vi "SCPI.vi"(4 "error in":T13, 7 "Command":string) -> (0 "error out":T13, 3 "Response":T11)   [LabVIEW 2018]
uses:
  MOKO_LabViewLibrary/MokoLowLevel/MokoLowLovelControl/MLLC_Error.ctl
  MOKO_LabViewLibrary/MokoLowLevel/MokoLowLovelControl/MLLC_Mode.ctl
  MOKO_LabViewLibrary/MokoLowLevel/MokoLowLovelControl/MLLC_Response.ctl
  MOKO_LabViewLibrary/MokoLowLevel/MokoLowLovelControl/MLLC_ConnectCluster.ctl
  MOKO_LabViewLibrary/MokoLowLevel/MokoLowLovelControl/MLLC_InterfaceType.ctl
  MOKO_LabViewLibrary/MokoLowLevel/MokoLowLovelControl/MLLC_OpenedSession.ctl
  MOKO_LabViewLibrary/MokoLowLevel/MokoLowLovelControl/MLLC_InterfaceSettings.ctl
  MOKO_LabViewLibrary/MokoLowLevel/MokoLowLovelControl/MLLC_InterfaceKind.ctl
  MOKO_LabViewLibrary/MokoLowLevel/MokoLowLovelControl/MLLC_DriverName.ctl
  MOKO_LabViewLibrary/MokoLowLevel/MokoLowLovelControl/MLLC_ErrorCode.ctl
  MOKO_LabViewLibrary/MokoLowLevel/MokoLowLovelControl/MLLC_ResponseInit.ctl
  MOKO_LabViewLibrary/MokoLowLevel/MokoLowLovelControl/MLLC_Request.ctl
panel:
  in  "Request":T1="*IDN?"
  in  "Response Init":T2="SCPI"
  in  "Error Code":T3=5450
  in  "Driver Name":T4="SCPI"
  in  "Settings":T10={"Saved Data"=variant, "Permanent data"={"Connect"={"InterfaceType"=enum."VISA", "OpenedSession"="COM1", "InterfaceSettings"={"Interface"=enum."Ethernet", "EOS 4 read"=enum."LF (\\n)", "EOS 4 write"=enum."LF (\\n)", "TMO, ms"=10000, "Sett"=variant(cluster{"Baud Rate":u32, "Data Bits":u16, "Parity":u16, "Stop Bits":u16, "Flow Control":u16, "Eho":bool} {"Baud Rate"=75, "Data Bits"=0, "Parity"=0, "Stop Bits"=0, "Flow Control"=0, "Eho"=FALSE})}}}}
  in  "Mode":T12=enum."Check"
  # "Example SCPI"
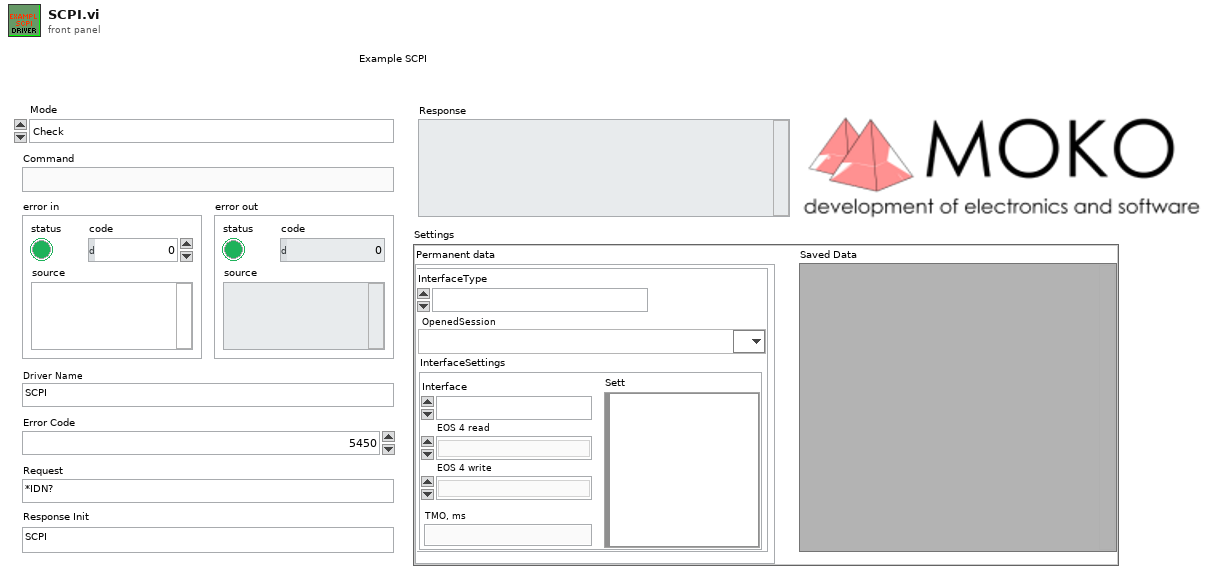
[diagram p1: front panel]
types:
  T1 = typedef "MLLC_Request.ctl" = string
  T2 = typedef "MLLC_ResponseInit.ctl" = string
  T3 = typedef "MLLC_ErrorCode.ctl" = u32
  T4 = typedef "MLLC_DriverName.ctl" = string
  T5 = typedef "MLLC_ConnectCluster.ctl" = cluster{"InterfaceType":T6, "OpenedSession":T7, "InterfaceSettings":T8}
  T6 = typedef "MLLC_InterfaceType.ctl" = enum16{"VISA", "Prologix USB-GPIB"}
  T7 = typedef "MLLC_OpenedSession.ctl" = refnum<visa-resource-name>
  T8 = typedef "MLLC_InterfaceSettings.ctl" = cluster{"Interface":T9, "EOS 4 read":enum16{"Default (=EOS 4 write)", "CR (\\r)", "LF (\\n)", "None"}, "EOS 4 write":enum16{"CR+LF (\\r\\n)", "CR (\\r)", "LF (\\n)", "None"}, "TMO, ms":i32, "Sett":variant}
  T9 = typedef "MLLC_InterfaceKind.ctl" = enum16{"RS232", "GPIB", "USB", "Ethernet", "another"}
  T10 = cluster{"Saved Data":variant, "Permanent data":cluster{"Connect":T5}}
  T11 = typedef "MLLC_Response.ctl" = string
  T12 = typedef "MLLC_Mode.ctl" = enum16{"get", "set", "close", "Init", "Check"}
  T13 = typedef "MLLC_Error.ctl" = errorcluster
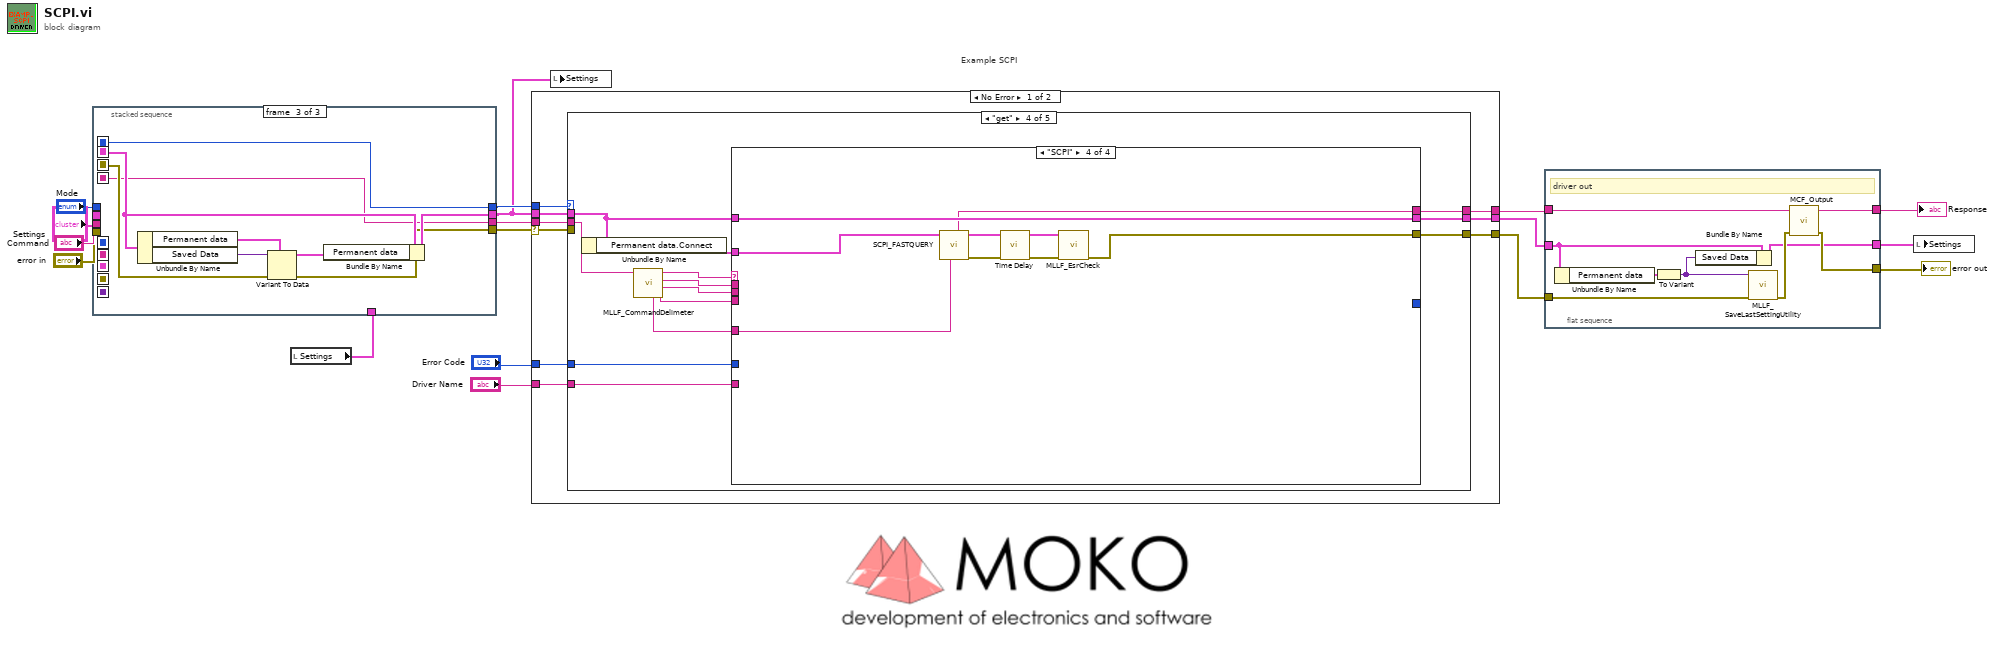
[diagram p0: block diagram]
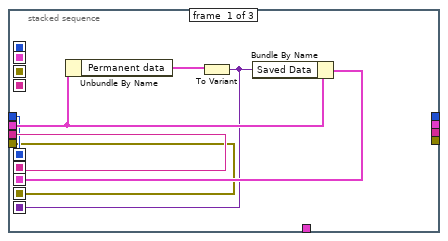
[diagram p2: hidden frame]
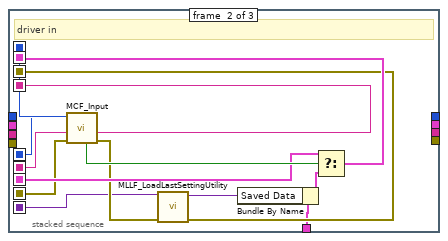
[diagram p3: hidden frame]
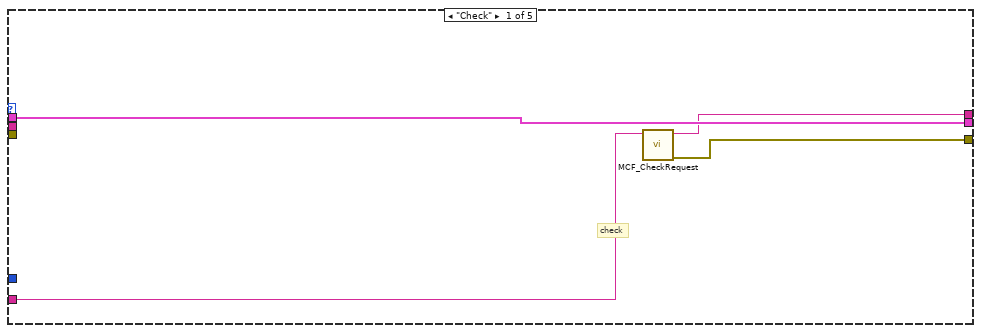
[diagram p4: hidden frame]
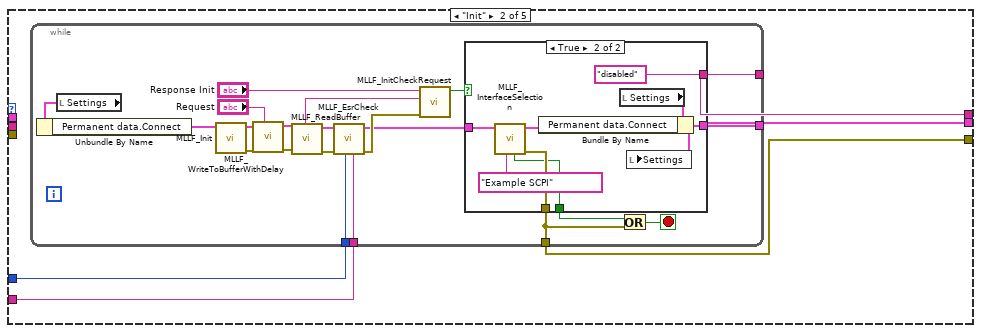
[diagram p5: hidden frame]
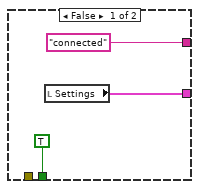
[diagram p6: hidden frame]
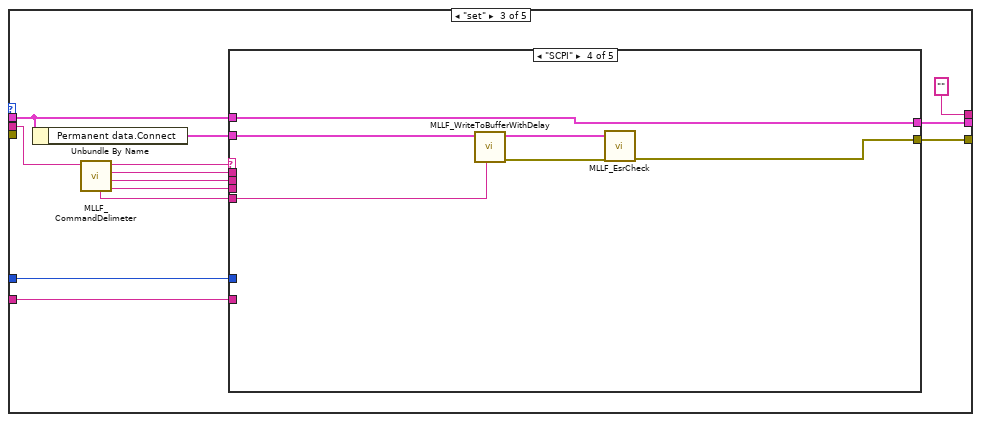
[diagram p7: hidden frame]
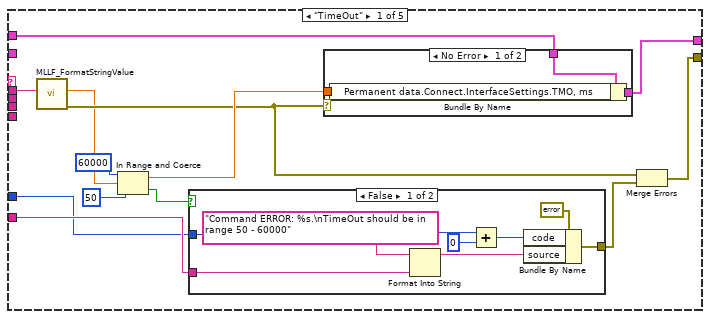
[diagram p8: hidden frame]
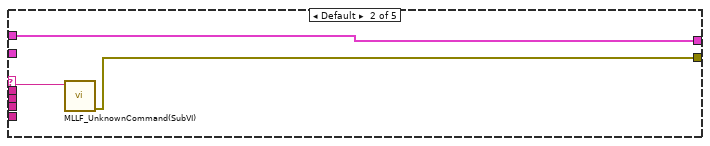
[diagram p11: hidden frame]
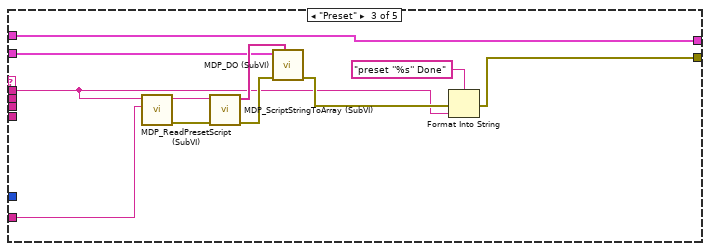
[diagram p12: hidden frame]
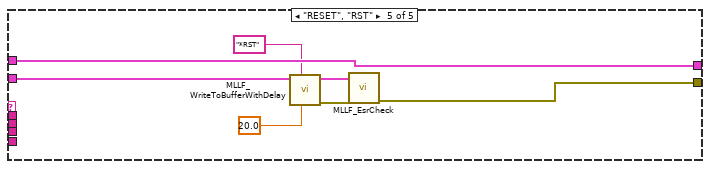
[diagram p13: hidden frame]
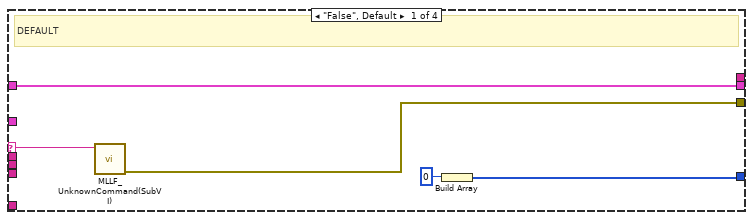
[diagram p14: hidden frame]
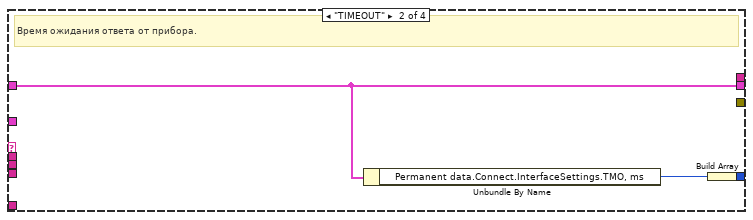
[diagram p15: hidden frame]
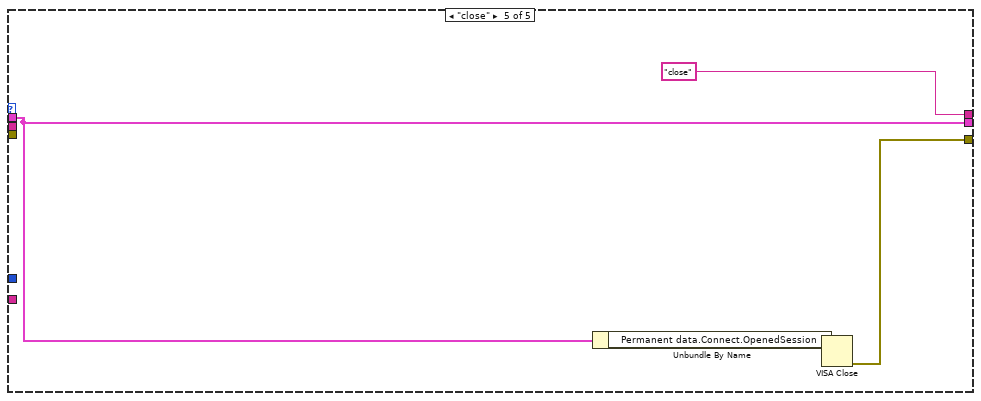
[diagram p17: hidden frame]
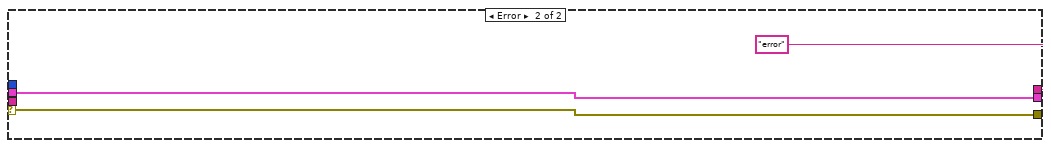
[diagram p18: hidden frame]
diagram:
  # "Example SCPI"
  n1 = local read "Settings"() -> (w7:T10)
  n2 = stacked-sequence {
    seq-local: [w20 _ _] -> [_ w36 _]
    seq-local: [w19 _ _] -> [_ w37 _]
    seq-local: [w22 _ _] -> [_ w32 _]
    seq-local: [w18 _ _] -> [_ w31 _]
    seq-local: [w21 _ _] -> [_ w27 _]
    seq-local: [_ w28 _] -> [_ _ w44]
    seq-local: [_ w38 _] -> [_ _ w41]
    seq-local: [_ w35 _] -> [_ _ w40]
    seq-local: [_ w34 _] -> [_ _ w45]
    tunnel: "Command" -> [w20 _ _]
    tunnel: "Mode" -> [w19 _ _]
    tunnel: "error in" -> [w18 _ _]
    tunnel: "Settings" -> [w23 _ _]
    tunnel: w7 -> [_ w26 _]
    tunnel: [_ _ w40] -> w9
    tunnel: [_ _ w43] -> w10
    tunnel: [_ _ w42] -> w8
    tunnel: [_ _ w41] -> w11
    frame #0 {
      n3 = Unbundle By Name(w23) -> ("Permanent data"=w24:cluster{"Connect":T5})
      n4 = To Variant(anything=w24) -> (Variant=w21:variant)
      n5 = Bundle By Name(cluster=w23, "Saved Data"=w21) -> (w22:T10)
    }
    frame #1 {
      # "driver in"
      n6 = call "MCF_Input.vi"("Error In"=w31, "Command in"=w36, "Mode in"=w37) -> ("Error Out"=w30:errorcluster, "Command out"=w35:string, "Mode out"=w38:T12, "Boolean"=w33:bool)  [unwired: 5 in]
      n7 = call "MLLF_LoadLastSettingUtility.vi"("Error In"=w30, "Save data in"=w27) -> ("Error Out"=w28:errorcluster, "Save data out"=w25:variant)  [unwired: 8 in]
      n8 = Bundle By Name(cluster=w26, "Saved Data"=w25) -> (w29:T10)
      n9 = Select(t=w32, s=w33, f=w29) -> (s? t:f=w34:T10)
    }
    frame #2 {
      n10 = Unbundle By Name(w45) -> ("Permanent data"=w46:cluster{"Connect":T5}, "Saved Data"=w39:variant)
      n11 = Variant To Data(error in=w44, type=w46, Variant=w39) -> (data=w47:cluster{"Connect":T5}, error out=w42:errorcluster)
      n12 = Bundle By Name(cluster=w45, "Permanent data"=w47) -> (w43:T10)
    }
  }
  n13 = case shown="No Error" w8 {
    selector: w8 -> [w52 w199]
    tunnel: [w54 w199] -> w4
    tunnel: w11 -> [w56 _]
    tunnel: [w55 "error" ("Output String")] -> w6
    tunnel: w9 -> [w53 _]
    tunnel: w10 -> [w49 w198]
    tunnel: "Error Code" -> [w51 _]
    tunnel: "Driver Name" -> [w50 _]
    tunnel: [w48 w198] -> w5
    frame No Error {
      n14 = case shown="\"get\"" w56 {
        tunnel: [w58 w63 "" ("Output String") w167 "close" ("Output String")] -> w55
        tunnel: [w57 w62 w103 w169 w195] -> w54
        tunnel: w53 -> [_ _ w110 w175 _]
        tunnel: w52 -> [_ _ _ _ _]
        tunnel: w51 -> [_ w65 w109 w172 _]
        tunnel: w50 -> [w59 w64 w106 w171 _]
        tunnel: w49 -> [w60 _ w108 w174 w194]
        tunnel: [w60 w61 w107 w173 w194] -> w48
        frame "Check" {
          # "check"
          # "Проверка подленности пользователя в соответствии с протоколом MD5."
          n15 = call "MCF_CheckRequest.vi"("Driver Name"=w59) -> ("Error Out"=w57:errorcluster, "Output String"=w58:string)  [unwired: 9 in]
        }
        frame "Init" {
          # "Тут проходит инициализация оборудования"
          n16 = while {
            tunnel: [w79] -> w62
            tunnel: w65 -> [w71]
            tunnel: w64 -> [w70]
            tunnel: [w76] -> w63
            tunnel: [w77] -> w61
            stop <- w78 stop-if-true
            n17 = local read "Settings"() -> (w82:T10)
            n18 = Unbundle By Name(w82) -> ("Permanent data.Connect"=w73:T5)
            n19 = call "MLLF_Init.vi"("DriverConnect in"=w73) -> ("Error Out"=w84:errorcluster, "DriverConnect out"=w83:T5)  [unwired: 7 in]
            n20 = call "MLLF_WriteToBufferWithDelay.vi"("Command"="Request", "Error In"=w84, "DriverConnect in"=w83) -> ("Error Out"=w86:errorcluster, "DriverConnect out"=w85:T5)  [unwired: 7 in]
            n21 = call "MLLF_ReadBuffer.vi"("Error In"=w86, "DriverConnect in"=w85) -> ("Error Out"=w68:errorcluster, "DriverConnect out"=w69:T5, "String"=w75:string)  [unwired: 6 in]
            n22 = call "MLLF_EsrCheck.vi"("Name"=w70, "Error code"=w71, "error in"=w68, "DriverConnect in"=w69) -> ("error out"=w67:T13, "DriverConnect out"=w66:T5)  [unwired: 6 in]
            n23 = call "MLLF_InitCheckRequest.vi"("error in (no error)"=w67, "Answer"=w75, "Response Init"="Response Init") -> ("Design"=w72:bool)  [unwired: 5 in, 3 out]
            n24 = case shown="True" w72 {
              tunnel: w66 -> [_ w96]
              tunnel: [TRUE w90] -> w80
              tunnel: [_ w97] -> w79
              tunnel: [w88 w92] -> w77
              tunnel: ["connected" "disabled"] -> w76
              frame False {
                n25 = local read "Settings"() -> (w88:T10)
              }
              frame True {
                n26 = call "MLLF_InterfaceSelection.vi"("Driver Name"="Example SCPI" ("String"), "DriverConnect in"=w96) -> ("error out"=w97:T13, "DriverConnect out"=w94:T5, "stop init?"=w90:bool)  [unwired: 7 in]
                n27 = local read "Settings"() -> (w93:T10)
                n28 = Bundle By Name(cluster=w93, "Permanent data.Connect"=w94) -> (w92:T10)
                n29 = local write "Settings"(w92) -> ()
              }
            }
            n30 = Or(x=w80, y=w79) -> (x .or. y?=w78:bool)
          }
        }
        frame "set" {
          # "Тут реализованы функции DriverSet"
          n31 = Unbundle By Name(w108) -> ("Permanent data.Connect"=w104:T5)
          n32 = call "MLLF_CommandDelimeter.vi"("command with param"=w110) -> ("param 3"=w99:string, "param 2"=w100:string, "param 1"=w101:string, "command"=w102:string, "Spit delimetre"=w98:string)  [unwired: 6 in]
          n33 = case shown="\"SCPI\"" w102 {
            selector: w102 -> [_ w137 _ _ _]
            tunnel: w108 -> [w113 w138 w139 w154 w162]
            tunnel: [w112 w138 w139 w154 w162] -> w107
            tunnel: w101 -> [w111 _ w142 _ _]
            tunnel: w109 -> [w115 _ _ _ _]
            tunnel: w106 -> [w116 _ w141 _ _]
            tunnel: [w114 w136 w140 w153 w161] -> w103
            tunnel: w104 -> [_ _ w143 w155 w160]
            tunnel: w100 -> [_ _ _ _ _]
            tunnel: w99 -> [_ _ _ _ _]
            tunnel: w98 -> [_ _ _ w150 _]
            frame "TimeOut" {
              n34 = call "MLLF_FormatStringValue.vi"("String Value"=w111) -> ("error out"=w118:T13, "number"=w117:dbl)  [unwired: 8 in, 1 out]
              n35 = In Range and Coerce(upper limit=60000, x=w117, lower limit=50) -> (coerced(x)=w121:dbl, In Range?=w119:bool)
              n36 = case shown="False" w119 {
                tunnel: [w130 _] -> w120
                tunnel: w115 -> [w129 _]
                tunnel: w116 -> [w128 _]
                frame False {
                  n37 = Format Into String(format string="Command ERROR: %s.\nTimeOut should be in range 50 - 60000", w128) -> (resulting string=w132:string)  [unwired: 2 in, 1 out]
                  n38 = Add(x=w129, y=0) -> (x+y=w133:T3)
                  n39 = Bundle By Name(cluster=errorcluster {"status"=TRUE, "code"=0, "source"=""} ("error out"), "code"=w133, "source"=w132) -> (w130:errorcluster)
                }
                frame True {
                }
              }
              n40 = case shown="No Error" w118 {
                tunnel: [w126 w127] -> w112
                tunnel: w113 -> [w125 w127]
                tunnel: w121 -> [w124 _]
                frame No Error {
                  n41 = Bundle By Name(cluster=w125, "Permanent data.Connect.InterfaceSettings.TMO, ms"=w124) -> (w126:T10)
                }
                frame Error {
                }
              }
              n42 = Merge Errors(w118, w120) -> (w114:errorcluster)
            }
            frame Default {
              n43 = call "MLLF_UnknownCommand(SubVI).vi"("Unknown command"=w137) -> ("error out"=w136:errorcluster)  [unwired: 10 in]
            }
            frame "Preset" {
              n44 = call "MDP_ReadPresetScript (SubVI).vi"("Driver Name"=w141, "String in"=w142) -> ("Error Out"=w147:errorcluster, "String out"=w148:string)  [unwired: 8 in]
              n45 = call "MDP_ScriptStringToArray (SubVI).vi"("Error In"=w147, "String script"=w148) -> ("Error Out"=w149:errorcluster, "Array script"=w144:string[])  [unwired: 8 in]
              n46 = call "MDP_DO (SubVI).vi"("Array script"=w144, "Error in (no error)"=w149, "DriverConnect in"=w143) -> ("Error Out"=w145:errorcluster)  [unwired: 7 in, 1 out]
              n47 = Format Into String(format string="preset ''%s'' Done" ("Befor substring"), error in=w145, w142) -> (error out=w140:errorcluster)  [unwired: 1 in, 1 out]
            }
            frame "SCPI" {
              n48 = call "MLLF_WriteToBufferWithDelay.vi"("Command"=w150, "DriverConnect in"=w155) -> ("Error Out"=w151:errorcluster, "DriverConnect out"=w152:T5)  [unwired: 8 in]
              n49 = call "MLLF_EsrCheck.vi"("error in"=w151, "DriverConnect in"=w152) -> ("error out"=w153:T13)  [unwired: 8 in, 1 out]
            }
            frame "RESET", "RST" {
              n50 = call "MLLF_WriteToBufferWithDelay.vi"("Delay Time ( 0,05 s)"=20.0, "Command"="*RST" ("string"), "DriverConnect in"=w160) -> ("Error Out"=w158:errorcluster, "DriverConnect out"=w157:T5)  [unwired: 7 in]
              n51 = call "MLLF_EsrCheck.vi"("error in"=w158, "DriverConnect in"=w157) -> ("error out"=w161:T13)  [unwired: 8 in, 1 out]
            }
          }
        }
        frame "get" {
          # "Тут реализованы функции DriverGet"
          n52 = Unbundle By Name(w174) -> ("Permanent data.Connect"=w170:T5)
          n53 = call "MLLF_CommandDelimeter.vi"("command with param"=w175) -> ("param 3"=w164:string, "param 2"=w165:string, "param 1"=w166:string, "command"=w168:string, "Spit delimetre"=w163:string)  [unwired: 6 in]
          n54 = case shown="\"SCPI\"" w168 {
            selector: w168 -> [w177 _ _ _]
            tunnel: [w176 _ _ w189] -> w169
            tunnel: w172 -> [_ _ _ _]
            tunnel: [w180 w183 w184 w191] -> w173
            tunnel: w174 -> [w180 w183 w184 w191]
            tunnel: [w178 w181 _ _] -> _
            tunnel: w170 -> [_ _ _ w192]
            tunnel: w171 -> [_ _ _ _]
            tunnel: [_ _ _ w188] -> w167
            tunnel: w166 -> [_ _ _ _]
            tunnel: w165 -> [_ _ _ _]
            tunnel: w164 -> [_ _ _ _]
            tunnel: w163 -> [_ _ _ w185]
            frame "False", Default {
              # "DEFAULT"
              n55 = call "MLLF_UnknownCommand(SubVI).vi"("Unknown command"=w177) -> ("error out"=w176:errorcluster)  [unwired: 10 in]
              n56 = Build Array(0 ("TimeOut")) -> (w178:i32[])
            }
            frame "TIMEOUT" {
              # "Время ожидания ответа от прибора."
              n57 = Unbundle By Name(w183) -> ("Permanent data.Connect.InterfaceSettings.TMO, ms"=w182:i32)
              n58 = Build Array(w182) -> (w181:i32[])
            }
            frame "------ID-------" {
            }
            frame "SCPI" {
              n59 = call "SCPI_FASTQUERY.vi"("input"=w185, "DriverConnect in"=w192) -> ("error out"=w187:T13, "DriverConnect out"=w190:T5, "output"=w188:string)  [unwired: 7 in]
              n60 = call "Time Delay"("error in (no error)"=w187) -> ("error out"=w186:errorcluster)  [unwired: 10 in]
              n61 = call "MLLF_EsrCheck.vi"("error in"=w186, "DriverConnect in"=w190) -> ("error out"=w189:T13)  [unwired: 8 in, 1 out]
            }
          }
        }
        frame "close" {
          # "Завершение сессии"
          n62 = Unbundle By Name(w194) -> ("Permanent data.Connect.OpenedSession"=w196:T7)
          n63 = VISA Close(VISA resource name=w196) -> (error out=w195:errorcluster)  [unwired: 1 in]
        }
      }
    }
    frame Error {
    }
  }
  n64 = local write "Settings"(w10) -> ()
  n65 = flat-sequence {
    tunnel: [w208] -> w3
    tunnel: [w207] -> w2
    tunnel: w6 -> [w206]
    tunnel: w4 -> [w205]
    tunnel: w5 -> [w201]
    tunnel: [w203] -> w1
    frame #0 {
      # "driver out"
      n66 = Unbundle By Name(w201) -> ("Permanent data"=w200:cluster{"Connect":T5})
      n67 = To Variant(anything=w200) -> (Variant=w202:variant)
      n68 = Bundle By Name(cluster=w201, "Saved Data"=w202) -> (w203:T10)
      n69 = call "MLLF_SaveLastSettingUtility.vi"("error in"=w205, "Saved Data"=w202) -> ("error out"=w204:T13)  [unwired: 8 in, 1 out]
      n70 = call "MCF_Output.vi"("Error In"=w204, "Input"=w206) -> ("Error Out"=w207:errorcluster, "Output"=w208:string)  [unwired: 8 in]
    }
  }
  n71 = local write "Settings"(w1) -> ()
  "error out" <- w2
  "Response" <- w3
